vi "PQgetResult.vi"(8 "error in (no error)":errorcluster, 11 "conn":u32) -> (0 "error out":errorcluster, 2 "PGresult":u32, 3 "conn_out":u32)   [LabVIEW 2019, in "libpqlv.lvlib"]
doc: "Waits for the next result from a prior PQsendQuery, PQsendQueryParams, PQsendPrepare, or PQsendQueryPrepared call, and returns it. A null pointer is returned when the command is complete and there will be no more results.\n\n PGresult *PQgetResult(PGconn *conn);\nhttp://www.postgresql.org/docs/8.3/static/libpq-async.html"
uses:
  libpqlv.lvlib
  libpq.dll
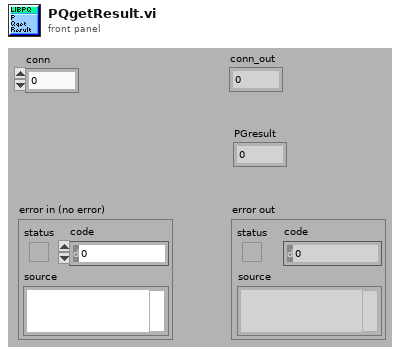
[diagram p1: front panel]
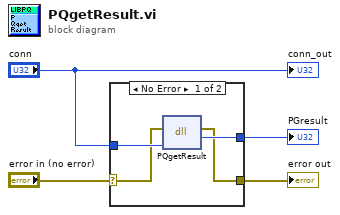
[diagram p0: block diagram]
diagram:
  n1 = case shown="No Error" "error in (no error)" {
    selector: "error in (no error)" -> [w6 w9]
    tunnel: [w5 w9] -> w2
    tunnel: "conn" -> [w8 _]
    tunnel: [w7 _] -> w4
    frame No Error {
      n2 = dll-call lib="libpq.*" fn="PQgetResult"(error in=w6, "conn"=w8) -> (error out=w5:errorcluster, "PGresult"=w7:u32)  [unwired: 3 in, 1 out]
    }
    frame Error {
    }
  }
  "PGresult" <- w4
  "error out" <- w2
  "conn_out" <- "conn"
